vi "Pressure_1_R3.vi"() -> ()   [LabVIEW 2020]
uses:
  Support/Controls/Cmd_Mouse Popup.ctl
  Support/Controls/Clst_Initialize Input.ctl
  Support/Controls/Cmd_Var Data IO.ctl
  Variables/Global_Cal Info.vi
panel:
  in  "Measured_ADJ":string[][](table) caption="Measured (조정후)"
  out "최소용량":string
  out "분동조합":string[][](table)
  out "Form":string[][](table)
  in  "교정방법":string(combo)="기본교정"
  out "Resolution":string[][](table) caption="Spec"
  in  "지시형태":string(combo)="Check"
  in  "Spec 변경":bool
  in  "Random":bool
  out "Spec":string[][](table)
  out "제목":string
  out "에러 출력":errorcluster
  out "Condition":string[][](table)
  in  "최소눈금":string(combo)
  out "단위":string
  out "최대용량":string
  in  "Measured":string[][](table)
  out "Load?":bool
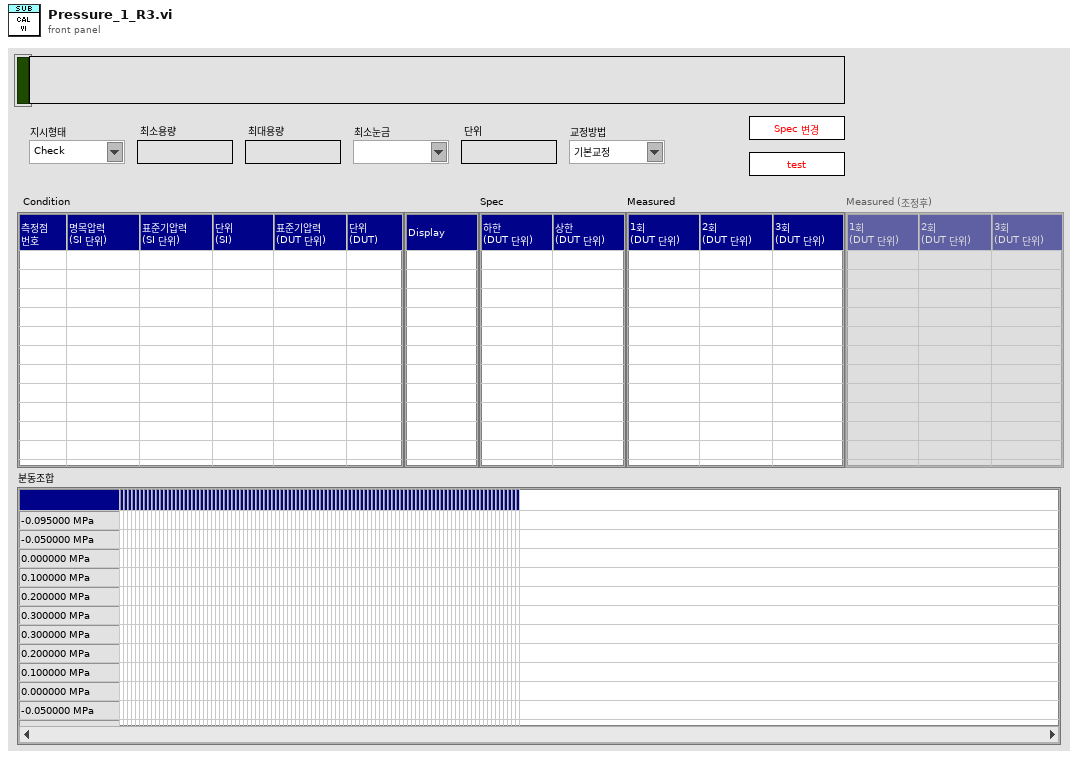
[diagram p1: front panel]
types:
  T1 = typedef "Cmd_Mouse Popup.ctl" = enum16{"활성화", "메뉴선택"}
  T2 = cluster{"Shift":bool, "Ctrl":bool, "Alt":bool, "Cmd":bool, "Opt":bool}
  T3 = typedef "Clst_Initialize Input.ctl" = cluster{"Initialize 1":cluster{"Condition":refnum<vi>[], "Spec":refnum<vi>[], "Measured":refnum<vi>[], "Resolution":refnum<vi>[], "Func_ext":string, "제목":refnum<vi>, "Measured_ADJ":refnum<vi>[]}, "Initialize 2":cluster{"문자열":refnum<vi>[], "콤보박스":refnum<vi>[], "링":refnum<vi>[], "열거형":refnum<vi>[], "테이블":refnum<vi>[], "여러열":refnum<vi>[], "디지털(DBL)":refnum<vi>[], "3D string":refnum<vi>[], "ctrl":refnum<vi>[], "boolean":refnum<vi>[]}}
  T4 = typedef "Cmd_Var Data IO.ctl" = enum16{"Condition", "Condition Default", "Condition_Temp", "Resolution", "Resolution Default", "Resolution Old", "Spec", "Spec Default", "Spec Old", "Spec Temp", "Result", "Result2", "Result3", "Result_Temp", "Result_ADJ", "Result_ADJ2", "STD1", "STD2", "STD3", "STD4", "STD5", "STD Temp", "CMC", "CMC Default"}
  T5 = enum8{"Enabled", "Disabled", "Disabled and Grayed Out"}
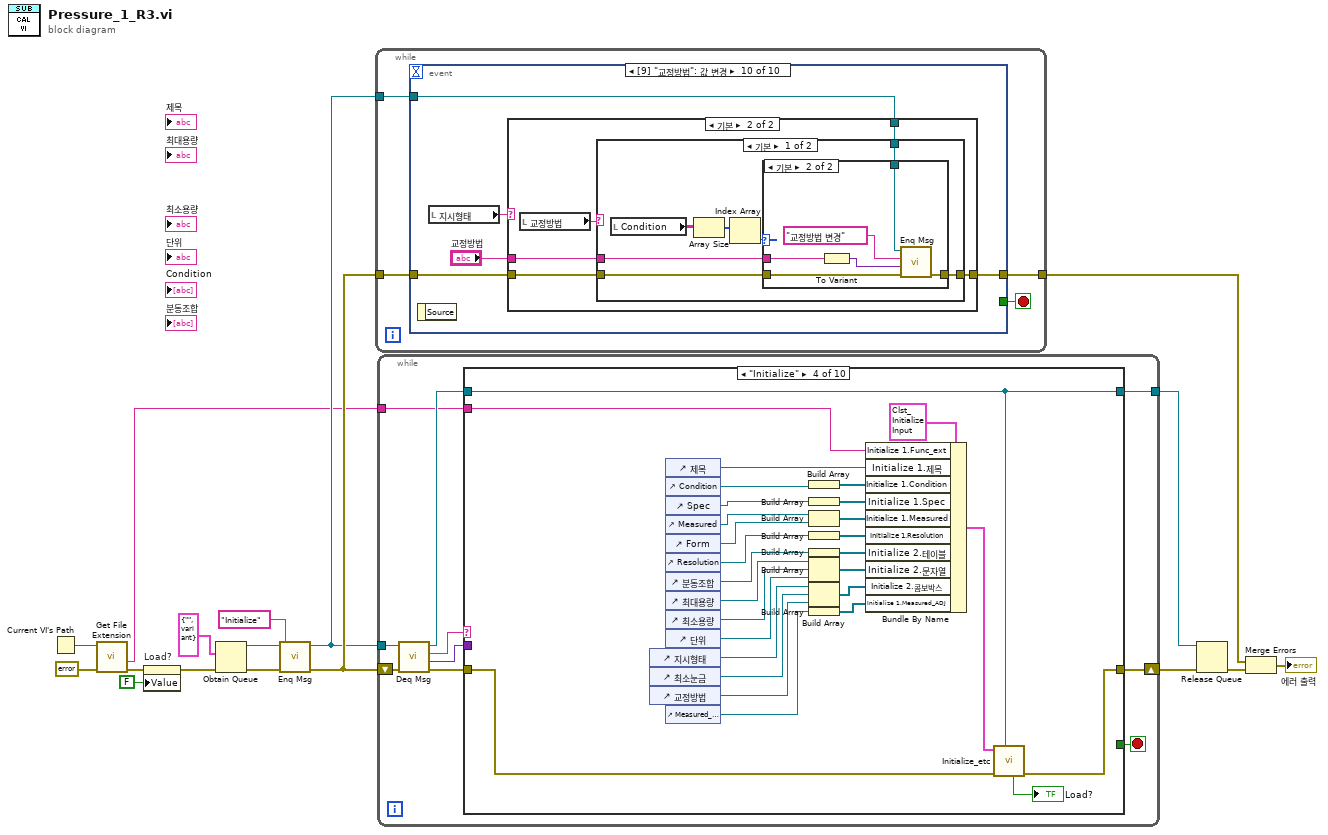
[diagram p0: block diagram]
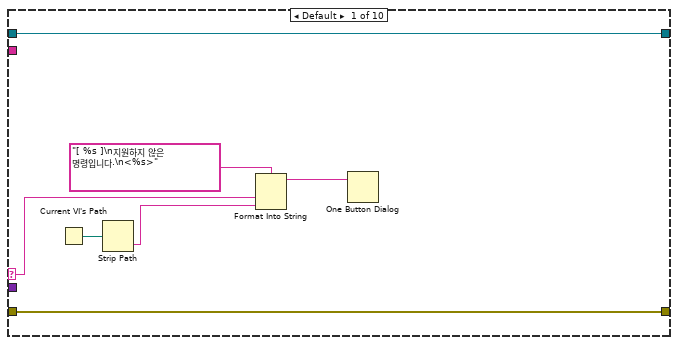
[diagram p2: hidden frame]
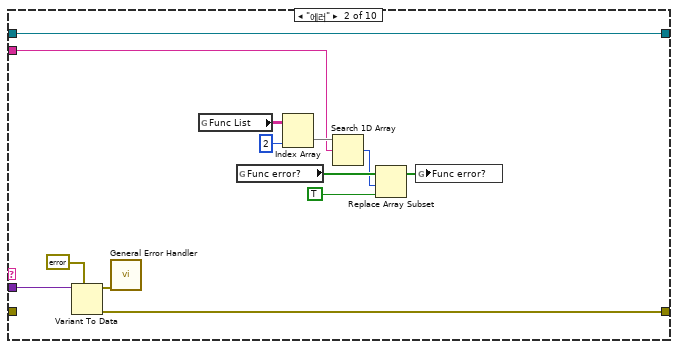
[diagram p3: hidden frame]
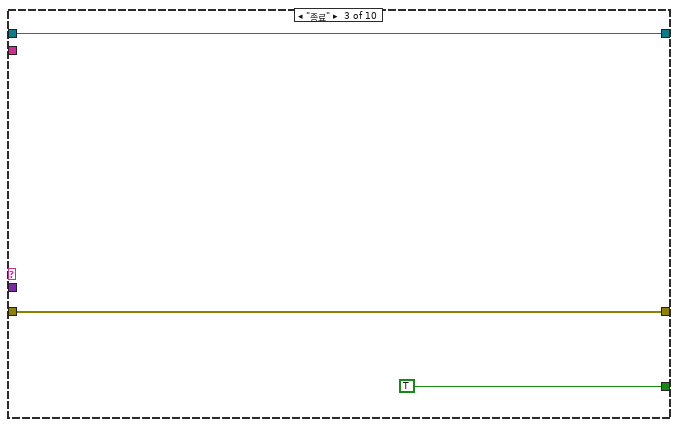
[diagram p4: hidden frame]
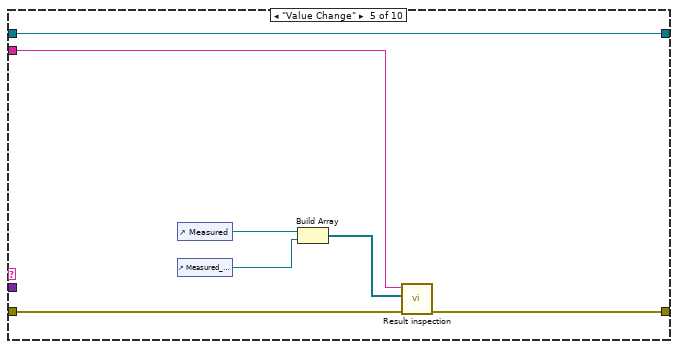
[diagram p5: hidden frame]
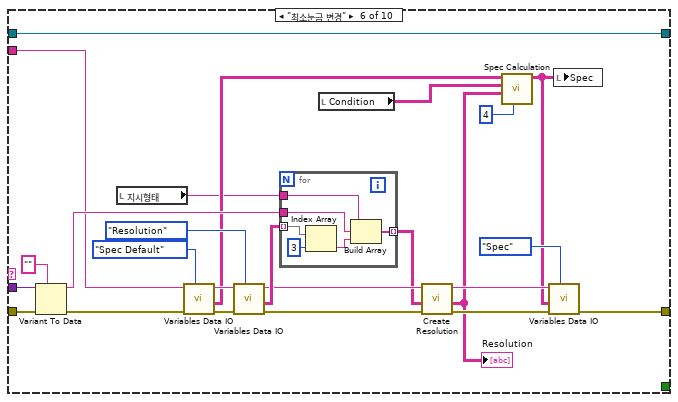
[diagram p6: hidden frame]
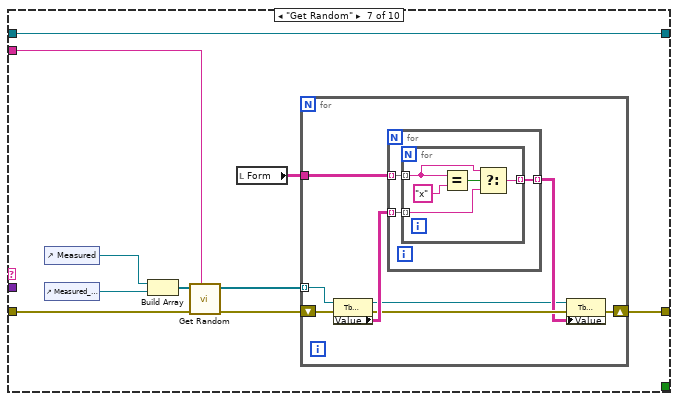
[diagram p7: hidden frame]
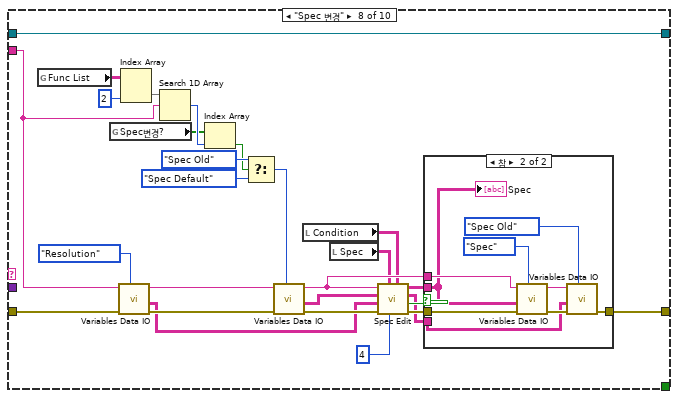
[diagram p8: hidden frame]
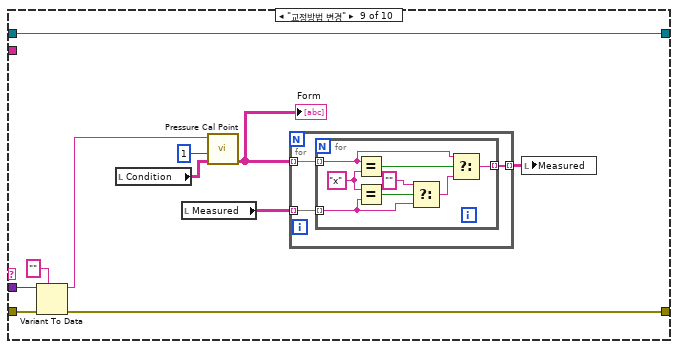
[diagram p10: hidden frame]
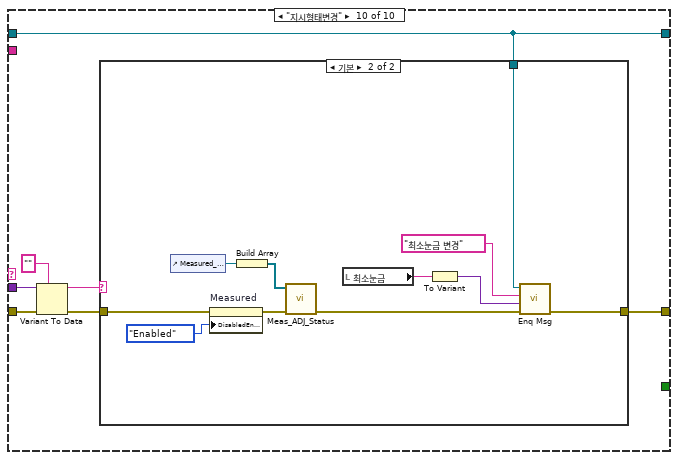
[diagram p11: hidden frame]
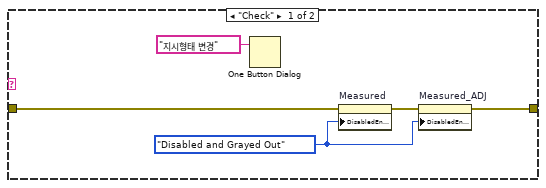
[diagram p12: hidden frame]
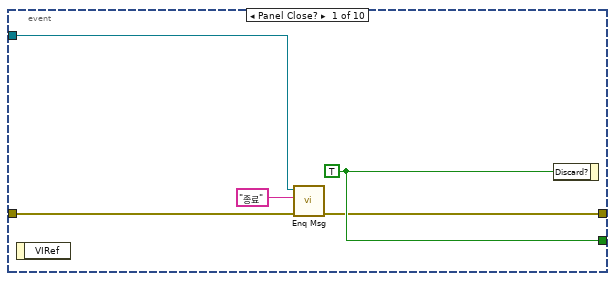
[diagram p13: hidden frame]
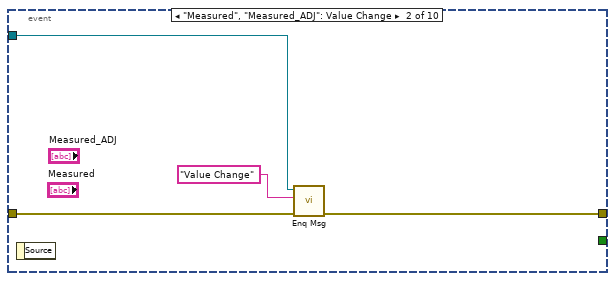
[diagram p14: hidden frame]
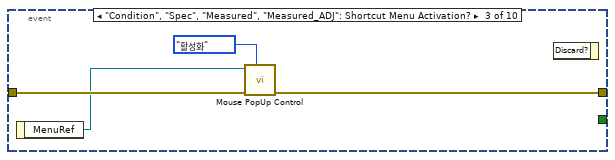
[diagram p15: hidden frame]
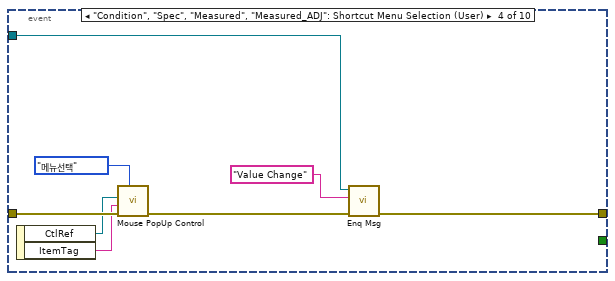
[diagram p16: hidden frame]
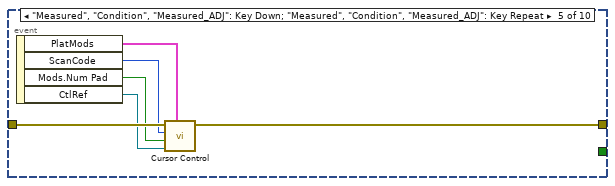
[diagram p17: hidden frame]
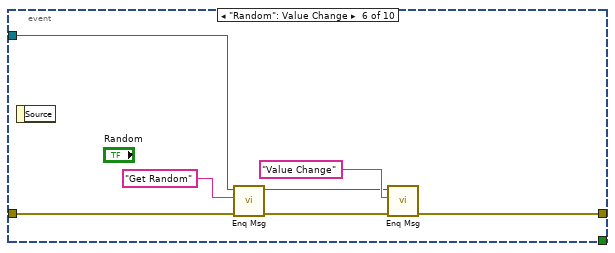
[diagram p18: hidden frame]
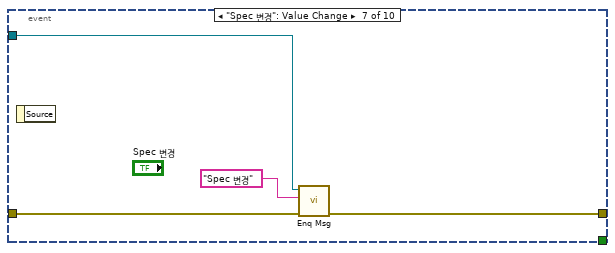
[diagram p19: hidden frame]
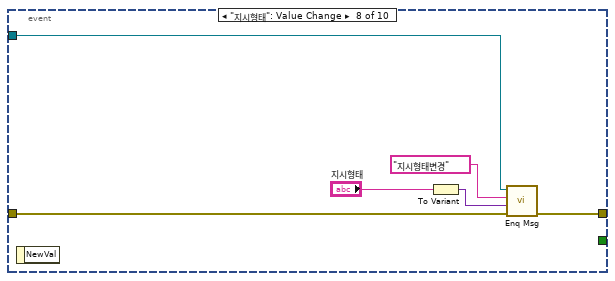
[diagram p20: hidden frame]
diagram:
  n1 = Current VI's Path() -> (path=w5:path)
  n2 = call <vilib>:"Get File Extension.vi"("error in (no error)"=errorcluster {"status"=FALSE, "code"=0, "source"=""} ("에러 상수"), "file"=w5) -> ("error out"=w3:errorcluster, "filename without extension"=w4:string)  [unwired: 5 in, 3 out]
  n3 = property on="Load?" class="Bool (엄격한)"(error in=w3, "Value"=FALSE ("Load?")) -> (error out=w2:errorcluster)  [unwired: 1 in, 1 out]
  n4 = Obtain Queue(element data type=cluster{"메세지":string, "값":variant} {"메세지"="", "값"=variant} ("Message Cluster"), error in (no error)=w2) -> (queue out=w14:refnum<queue>, error out=w16:errorcluster)  [unwired: 3 in, 1 out]
  n5 = call "Enq Msg.vi"("에러 입력(에러 없음)"=w16, "메세지"="Initialize", "큐 입력"=w14) -> ("에러 출력"=w15:errorcluster, "큐 출력"=w12:refnum<queue>)  [unwired: 7 in]
  n6 = while {
    tunnel: w15 -> [w19]
    tunnel: w12 -> [w20]
    tunnel: [w18] -> w9
    stop <- w21 stop-if-true
    n7 = event shown="[9] \"교정방법\": 값 변경" {
      selector: _ -> [_ _ _ _ _ _ _ _ _ _]
      dyn-events: _ -> [_ _ _ _ _ _ _ _ _ _]
      timeout: _ -> [_ _ _ _ _ _ _ _ _ _]
      tunnel: [w26 _ _ _ _ _ _ _ _ _] -> w21
      tunnel: w20 -> [w24 w29 _ w37 _ w50 w56 w62 w70 w72]
      tunnel: w19 -> [w25 w30 w33 w41 w48 w51 w58 w64 w71 w75]
      tunnel: [w22 w28 w32 w36 w47 w49 w57 w63 w69 w76] -> w18
      event Panel Close? {
        w26 = TRUE ("버림?")
        n8 = event-data() -> ()  [unwired: 1 in, 1 out]
        n9 = call "Enq Msg.vi"("에러 입력(에러 없음)"=w25, "메세지"="종료", "큐 입력"=w24) -> ("에러 출력"=w22:errorcluster)  [unwired: 7 in, 1 out]
        n10 = event-data("Discard?"=w26) -> ()  [unwired: 1 in, 1 out]
      }
      event "Measured", "Measured_ADJ": Value Change {
        n11 = event-data() -> ()  [unwired: 1 in, 1 out]
        n12 = call "Enq Msg.vi"("에러 입력(에러 없음)"=w30, "메세지"="Value Change", "큐 입력"=w29) -> ("에러 출력"=w28:errorcluster)  [unwired: 7 in, 1 out]
      }
      event "Condition", "Spec", "Measured", "Measured_ADJ": Shortcut Menu Activation? {
        n13 = event-data() -> ("MenuRef"=w31:refnum<k9>)  [unwired: 1 in]
        n14 = call "Mouse PopUp Control.vi"("type"=Cmd_Mouse_Popup."활성화", "error in"=w33, "메뉴 참조"=w31) -> ("error out"=w32:errorcluster)  [unwired: 8 in]
        n15 = event-data() -> ()  [unwired: 2 in, 1 out]
      }
      event "Condition", "Spec", "Measured", "Measured_ADJ": Shortcut Menu Selection (User) {
        n16 = event-data() -> ("CtlRef"=w39:refnum<vi>, "ItemTag"=w40:string)  [unwired: 1 in]
        n17 = call "Mouse PopUp Control.vi"("type"=Cmd_Mouse_Popup."메뉴선택", "error in"=w41, "아이템 태그"=w40, "Tbl 참조 번호"=w39) -> ("error out"=w38:errorcluster)  [unwired: 7 in]
        n18 = call "Enq Msg.vi"("에러 입력(에러 없음)"=w38, "메세지"="Value Change", "큐 입력"=w37) -> ("에러 출력"=w36:errorcluster)  [unwired: 7 in, 1 out]
      }
      event "Measured", "Condition", "Measured_ADJ": Key Down; "Measured", "Condition", "Measured_ADJ": Key Repeat {
        n19 = event-data() -> ("PlatMods"=w43:T2, "ScanCode"=w46:i16, "Mods.Num Pad"=w45:bool, "CtlRef"=w44:refnum<vi>)  [unwired: 1 in]
        n20 = call "Cursor Control.vi"("플랫폼 조합키"=w43, "참조"=w44, "Num Pad"=w45, "ScanCode"=w46, "error in"=w48) -> ("error out"=w47:errorcluster)  [unwired: 5 in, 1 out]
      }
      event "Random": Value Change {
        n21 = event-data() -> ()  [unwired: 1 in, 1 out]
        n22 = call "Enq Msg.vi"("에러 입력(에러 없음)"=w51, "메세지"="Get Random", "큐 입력"=w50) -> ("에러 출력"=w53:errorcluster, "큐 출력"=w54:refnum<queue>)  [unwired: 7 in]
        n23 = call "Enq Msg.vi"("에러 입력(에러 없음)"=w53, "메세지"="Value Change", "큐 입력"=w54) -> ("에러 출력"=w49:errorcluster)  [unwired: 7 in, 1 out]
      }
      event "Spec 변경": Value Change {
        n24 = event-data() -> ()  [unwired: 1 in, 1 out]
        n25 = call "Enq Msg.vi"("에러 입력(에러 없음)"=w58, "메세지"="Spec 변경", "큐 입력"=w56) -> ("에러 출력"=w57:errorcluster)  [unwired: 7 in, 1 out]
      }
      event "지시형태": Value Change {
        n26 = event-data() -> ()  [unwired: 1 in, 1 out]
        n27 = To Variant(anything="지시형태") -> (Variant=w60:variant)
        n28 = call "Enq Msg.vi"("에러 입력(에러 없음)"=w64, "값"=w60, "메세지"="지시형태변경", "큐 입력"=w62) -> ("에러 출력"=w63:errorcluster)  [unwired: 6 in, 1 out]
      }
      event "최소눈금": Value Change {
        n29 = event-data() -> ()  [unwired: 1 in, 1 out]
        n30 = To Variant(anything="최소눈금") -> (Variant=w66:variant)
        n31 = call "Enq Msg.vi"("에러 입력(에러 없음)"=w71, "값"=w66, "메세지"="최소눈금 변경", "큐 입력"=w70) -> ("에러 출력"=w69:errorcluster)  [unwired: 6 in, 1 out]
      }
      event "교정방법": Value Change {
        n32 = event-data() -> ()  [unwired: 1 in, 1 out]
        n33 = local read "지시형태"() -> (w73:string)
        n34 = case shown="기본" w73 {
          tunnel: w75 -> [w78 w83]
          tunnel: w72 -> [_ w82]
          tunnel: [w78 w81] -> w76
          tunnel: "교정방법" -> [_ w80]
          frame "Check" {
            n35 = One Button Dialog(message="지시형태 변경" ("메시지")) -> ()  [unwired: 1 in, 1 out]
          }
          frame Default {
            n36 = local read "교정방법"() -> (w79:string)
            n37 = case shown="기본" w79 {
              tunnel: w83 -> [w90 w105]
              tunnel: w82 -> [w89 w104]
              tunnel: [w88 w103] -> w81
              tunnel: w80 -> [w87 w102]
              frame Default {
                n38 = local read "Condition"() -> (w84:string[][])
                n39 = Array Size(array=w84) -> (size(s)=w86:i32[])
                n40 = Index Array(array=w86) -> (element=w85:i32)  [unwired: 1 in]
                n41 = case shown="기본" w85 {
                  tunnel: w90 -> [w93 w99]
                  tunnel: w89 -> [_ w98]
                  tunnel: [w93 w96] -> w88
                  tunnel: w87 -> [_ w94]
                  frame 0..21 {
                    n42 = local write "교정방법"("기본교정" ("교정방법")) -> ()
                    n43 = One Button Dialog(message="표준, 종합 교정은 11 측정점 이상 가능" ("메시지")) -> ()  [unwired: 1 in, 1 out]
                  }
                  frame Default {
                    n44 = To Variant(anything=w94) -> (Variant=w95:variant)
                    n45 = call "Enq Msg.vi"("에러 입력(에러 없음)"=w99, "값"=w95, "메세지"="교정방법 변경", "큐 입력"=w98) -> ("에러 출력"=w96:errorcluster)  [unwired: 6 in, 1 out]
                  }
                }
              }
              frame "기본교정" {
                n46 = To Variant(anything=w102) -> (Variant=w100:variant)
                n47 = call "Enq Msg.vi"("에러 입력(에러 없음)"=w105, "값"=w100, "메세지"="교정방법 변경", "큐 입력"=w104) -> ("에러 출력"=w103:errorcluster)  [unwired: 6 in, 1 out]
              }
            }
          }
        }
      }
    }
  }
  n48 = while {
    shift-right: [w115] -> w11
    shift-left: w15 -> [w114]
    tunnel: w12 -> [w112]
    tunnel: [w107] -> w10
    tunnel: w4 -> [w106]
    stop <- w108 stop-if-true
    n49 = call "Deq Msg.vi"("에러 입력(에러 없음)"=w114, "큐 입력"=w112) -> ("에러 출력"=w113:errorcluster, "값"=w109:variant, "메세지"=w111:string, "큐 출력"=w110:refnum<queue>)  [unwired: 6 in]
    n50 = case shown="\"Initialize\"" w111 {
      selector: w111 -> [w118 _ _ _ _ _ _ _ _ _]
      tunnel: w113 -> [w122 _ w138 w151 w171 w197 w213 w252 w276 w296]
      tunnel: [w122 w132 w138 w140 w173 w179 w208 w256 w275 w297] -> w115
      tunnel: w110 -> [w121 w131 w136 w152 w174 w199 w215 w258 w279 w291]
      tunnel: w109 -> [_ w133 _ _ _ w196 _ _ w277 w294]
      tunnel: [_ _ TRUE ("버림?") _ _ _ _ _ _ _] -> w108
      tunnel: [w121 w131 w136 w152 w174 w199 w215 w258 w279 w291] -> w107
      tunnel: w106 -> [_ w123 _ w144 w172 w189 w211 w233 _ _]
      frame Default {
        n51 = Current VI's Path() -> (path=w117:path)
        n52 = Strip Path(path=w117) -> (name=w116:string)  [unwired: 1 out]
        n53 = Format Into String(format string="[ %s ]\n지원하지 않은 명령입니다.\n<%s>" ("메시지"), w118, w116) -> (resulting string=w119:string)  [unwired: 2 in, 1 out]
        n54 = One Button Dialog(message=w119) -> ()  [unwired: 1 in, 1 out]
      }
      frame "에러" {
        n55 = Variant To Data(type=errorcluster {"status"=FALSE, "code"=0, "source"=""} ("에러 출력"), Variant=w133) -> (data=w135:errorcluster, error out=w132:errorcluster)  [unwired: 1 in]
        n56 = call <vilib>:"General Error Handler.vi"("error in (no error)"=w135) -> ()  [unwired: 10 in, 5 out]
        n57 = global read "Global_Cal Info.vi" "Func List"() -> (w129:string[][])
        n58 = global read "Global_Cal Info.vi" "Func error?"() -> (w126:bool[])
        n59 = Index Array(array=w129, index (col)=2 ("비활성화된 인덱스 (열)")) -> (element=w128:string[])  [unwired: 1 in]
        n60 = Search 1D Array(1D array=w128, element=w123) -> (index of element=w125:i32)  [unwired: 1 in]
        n61 = Replace Array Subset(array=w126, new element=TRUE ("새 원소/부분배열"), index=w125) -> (w124:bool[])
        n62 = global write "Global_Cal Info.vi" "Func error?"(w124) -> ()
      }
      frame "종료" {
      }
      frame "Initialize" {
        n63 = control-ref of="지시형태"() -> (w147:refnum<vi>)
        n64 = control-ref of="최소눈금"() -> (w159:refnum<vi>)
        n65 = control-ref of="교정방법"() -> (w146:refnum<vi>)
        n66 = control-ref of="제목"() -> (w157:refnum<vi>)
        n67 = control-ref of="Condition"() -> (w165:refnum<vi>)
        n68 = control-ref of="Spec"() -> (w154:refnum<vi>)
        n69 = control-ref of="Measured"() -> (w162:refnum<vi>)
        n70 = control-ref of="Form"() -> (w145:refnum<vi>)
        n71 = control-ref of="Resolution"() -> (w149:refnum<vi>)
        n72 = control-ref of="분동조합"() -> (w150:refnum<vi>)
        n73 = control-ref of="최대용량"() -> (w156:refnum<vi>)
        n74 = control-ref of="최소용량"() -> (w143:refnum<vi>)
        n75 = control-ref of="단위"() -> (w155:refnum<vi>)
        n76 = control-ref of="Measured_ADJ"() -> (w142:refnum<vi>)
        n77 = Build Array(w165) -> (w164:refnum<vi>[])
        n78 = Build Array(w154) -> (w153:refnum<vi>[])
        n79 = Build Array(w162, w145) -> (w163:refnum<vi>[])
        n80 = Build Array(w149) -> (w148:refnum<vi>[])
        n81 = Build Array(w150) -> (w161:refnum<vi>[])
        n82 = Build Array(w156, w143, w155) -> (w160:refnum<vi>[])
        n83 = Build Array(w147, w159, w146) -> (w158:refnum<vi>[])
        n84 = Build Array(w142) -> (w141:refnum<vi>[])
        n85 = Bundle By Name(cluster=T3 {"Initialize 1"={"Condition"=[], "Spec"=[], "Measured"=[], "Resolution"=[], "Func_ext"="", "제목"=refnum, "Measured_ADJ"=[]}, "Initialize 2"={"문자열"=[], "콤보박스"=[], "링"=[], "열거형"=[], "테이블"=[], "여러열"=[], "디지털(DBL)"=[], "3D string"=[], "ctrl"=[], "boolean"=[]}} ("입력 클러스터"), "Initialize 1.Func_ext"=w144, "Initialize 1.제목"=w157, "Initialize 1.Condition"=w164, "Initialize 1.Spec"=w153, "Initialize 1.Measured"=w163, "Initialize 1.Resolution"=w148, "Initialize 2.테이블"=w161, "Initialize 2.문자열"=w160, "Initialize 2.콤보박스"=w158, "Initialize 1.Measured_ADJ"=w141) -> (w166:T3)
        n86 = call "Initialize_etc.vi"("큐 입력"=w152, "error in"=w151, "입력 클러스터"=w166) -> ("error out"=w140:errorcluster, "Load?"=→"Load?":bool)  [unwired: 6 in, 1 out]
      }
      frame "Value Change" {
        n87 = control-ref of="Measured"() -> (w170:refnum<vi>)
        n88 = control-ref of="Measured_ADJ"() -> (w168:refnum<vi>)
        n89 = Build Array(w170, w168) -> (w169:refnum<vi>[])
        n90 = call "Result inspection.vi"("error in"=w171, "Ref. Data (Inspection)"=w169, "Func ext"=w172) -> ("error out"=w173:errorcluster)  [unwired: 5 in, 3 out]
      }
      frame "최소눈금 변경" {
        n91 = Variant To Data(error in=w197, type="", Variant=w196) -> (data=w194:string, error out=w190:errorcluster)
        n92 = local read "지시형태"() -> (w175:string)
        n93 = call "Variables Data IO.vi"("Select"=Cmd_Var_Data_IO."Spec Default", "error in"=w190, "Func_ext"=w189) -> ("error out"=w187:errorcluster, "Data Out"=w185:string[][], "Func_ext Out"=w188:string)  [unwired: 6 in]
        n94 = call "Variables Data IO.vi"("Select"=Cmd_Var_Data_IO."Resolution", "error in"=w187, "Func_ext"=w188) -> ("error out"=w192:errorcluster, "Data Out"=w198:string[][], "Func_ext Out"=w191:string)  [unwired: 6 in]
        n95 = for {
          tunnel: w198 -> [w205] mode=indexing
          tunnel: w194 -> [w204]
          tunnel: [w202] -> w177 mode=indexing
          tunnel: w175 -> [w201]
          n96 = Index Array(array=w205, index=3 ("인덱스")) -> (element=w203:string)
          n97 = Build Array(w201, w204, w203) -> (w202:string[])
        }
        n98 = local read "Condition"() -> (w184:string[][])
        n99 = call "Create Resolution.vi"("에러 입력(에러 없음)"=w192, "Resolution"=w177, "Func_ext"=w191) -> ("에러 출력"=w180:errorcluster, "Resolution Out"=w176:string[][], "Func_ext 출력"=w181:string)  [unwired: 6 in]
        "Resolution" <- w176
        n100 = call "Spec Calculation.vi"("기준값 열번호"=4 ("열번호(기준값)"), "Resolution"=w176, "Condition in"=w184, "Spec Default"=w185) -> ("Spec out"=w178:string[][])  [unwired: 6 in, 1 out]
        n101 = call "Variables Data IO.vi"("Select"=Cmd_Var_Data_IO."Spec", "error in"=w180, "Data In"=w178, "Func_ext"=w181) -> ("error out"=w179:errorcluster)  [unwired: 5 in, 2 out]
        n102 = local write "Spec"(w178) -> ()
      }
      frame "Get Random" {
        n103 = control-ref of="Measured"() -> (w212:refnum<vi>)
        n104 = control-ref of="Measured_ADJ"() -> (w210:refnum<vi>)
        n105 = Build Array(w212, w210) -> (w214:refnum<vi>[])
        n106 = call "Get Random.vi"("Func_Ext"=w211, "에러 입력"=w213, "Meas"=w214) -> ("에러 출력"=w209:errorcluster, "Meas out"=w206:refnum<vi>[])  [unwired: 7 in]
        n107 = local read "Form"() -> (w207:string[][])
        n108 = for {
          tunnel: w207 -> [w222]
          shift-right: [w219] -> w208
          shift-left: w209 -> [w223]
          tunnel: w206 -> [w216] mode=indexing
          n109 = property on="프로퍼티 노드" class="Tbl (엄격한)"(reference=w216, error in=w223) -> (reference out=w217:refnum<vi>, error out=w220:errorcluster, "Value"=w221:string[][])
          n110 = for {
            tunnel: w222 -> [w226] mode=indexing
            tunnel: w221 -> [w225] mode=indexing
            tunnel: [w224] -> w218 mode=indexing
            n111 = for {
              tunnel: w226 -> [w229] mode=indexing
              tunnel: w225 -> [w228] mode=indexing
              tunnel: [w227] -> w224 mode=indexing
              n112 = Equal?(x=w229, y="ⅹ") -> (x = y?=w230:bool)
              n113 = Select(t=w229, s=w230, f=w228) -> (s? t:f=w227:string)
            }
          }
          n114 = property on="프로퍼티 노드" class="Tbl (엄격한)"(reference=w217, error in=w220, "Value"=w218) -> (error out=w219:errorcluster)  [unwired: 1 out]
        }
      }
      frame "Spec 변경" {
        n115 = global read "Global_Cal Info.vi" "Func List"() -> (w238:string[][])
        n116 = global read "Global_Cal Info.vi" "Spec변경?"() -> (w234:bool[])
        n117 = call "Variables Data IO.vi"("Select"=Cmd_Var_Data_IO."Resolution", "error in"=w252, "Func_ext"=w233) -> ("error out"=w251:errorcluster, "Data Out"=w245:string[][], "Func_ext Out"=w250:string)  [unwired: 6 in]
        n118 = Index Array(array=w238, index (col)=2 ("비활성화된 인덱스 (열)")) -> (element=w236:string[])  [unwired: 1 in]
        n119 = Search 1D Array(1D array=w236, element=w233) -> (index of element=w235:i32)  [unwired: 1 in]
        n120 = Index Array(array=w234, index=w235) -> (element=w239:bool)
        n121 = Select(t=Cmd_Var_Data_IO."Spec Old" ("Select"), s=w239, f=Cmd_Var_Data_IO."Spec Default" ("Select")) -> (s? t:f=w232:T4)
        n122 = call "Variables Data IO.vi"("Select"=w232, "error in"=w251, "Func_ext"=w250) -> ("error out"=w253:errorcluster, "Data Out"=w244:string[][], "Func_ext Out"=w246:string)  [unwired: 6 in]
        n123 = local read "Condition"() -> (w242:string[][])
        n124 = local read "Spec"() -> (w243:string[][])
        n125 = call "Spec Edit.vi"("Condition"=w242, "열번호(기준값)"=4 ("기준열(0)"), "Spec Value"=w243, "에러 입력(에러 없음)"=w253, "Resolution"=w245, "Spec Default"=w244, "Func_ext"=w246) -> ("에러 출력"=w257:errorcluster, "변경?"=w254:bool, "Spec Default out"=w248:string[][], "Spec 출력"=w255:string[][])  [unwired: 1 in]
        n126 = case shown="참" w254 {
          tunnel: w257 -> [w259 w267]
          tunnel: [w259 w263] -> w256
          tunnel: w255 -> [_ w265]
          tunnel: w246 -> [_ w266]
          tunnel: w248 -> [_ w261]
          frame False {
          }
          frame True {
            n127 = call "Variables Data IO.vi"("Select"=Cmd_Var_Data_IO."Spec", "error in"=w267, "Data In"=w265, "Func_ext"=w266) -> ("error out"=w264:errorcluster, "Func_ext Out"=w262:string)  [unwired: 5 in, 1 out]
            n128 = call "Variables Data IO.vi"("Select"=Cmd_Var_Data_IO."Spec Old", "error in"=w264, "Data In"=w261, "Func_ext"=w262) -> ("error out"=w263:errorcluster)  [unwired: 5 in, 2 out]
            "Spec" <- w265
          }
        }
      }
      frame "교정방법 변경" {
        n129 = Variant To Data(error in=w276, type="", Variant=w277) -> (data=w272:string, error out=w275:errorcluster)
        n130 = local read "Condition"() -> (w271:string[][])
        n131 = local read "Measured"() -> (w274:string[][])
        n132 = call "Pressure Cal Point.vi"("Condition"=w271, "인덱스 (열)"=1, "교정방법"=w272) -> ("배열"=w269:string[][])  [unwired: 5 in, 3 out]
        "Form" <- w269
        n133 = for {
          tunnel: w269 -> [w282] mode=indexing
          tunnel: w274 -> [w281] mode=indexing
          tunnel: [w280] -> w273 mode=indexing
          n134 = for {
            tunnel: w282 -> [w289] mode=indexing
            tunnel: w281 -> [w285] mode=indexing
            tunnel: [w283] -> w280 mode=indexing
            w288 = "ⅹ"
            n135 = Equal?(x=w289, y=w288) -> (x = y?=w290:bool)
            n136 = Equal?(x=w288, y=w285) -> (x = y?=w287:bool)
            n137 = Select(t="", s=w287, f=w285) -> (s? t:f=w284:string)
            n138 = Select(t=w289, s=w290, f=w284) -> (s? t:f=w283:string)
          }
        }
        n139 = local write "Measured"(w273) -> ()
      }
      frame "지시형태변경" {
        n140 = Variant To Data(error in=w296, type="", Variant=w294) -> (data=w292:string, error out=w295:errorcluster)
        n141 = case shown="기본" w292 {
          tunnel: w295 -> [w301 w312]
          tunnel: [w298 w305] -> w297
          tunnel: w291 -> [_ w303]
          frame "Check" {
            w300 = T5."Disabled and Grayed Out" ("비활성화")
            n142 = One Button Dialog(message="지시형태 변경" ("메시지")) -> ()  [unwired: 1 in, 1 out]
            n143 = property on="Measured" class="Tbl (엄격한)"(error in=w301, "DisabledEnum"=w300) -> (error out=w299:errorcluster)  [unwired: 1 in, 1 out]
            n144 = property on="Measured_ADJ" class="Tbl (엄격한)"(error in=w299, "DisabledEnum"=w300) -> (error out=w298:errorcluster)  [unwired: 1 in, 1 out]
          }
          frame Default {
            n145 = control-ref of="Measured_ADJ"() -> (w311:refnum<vi>)
            n146 = property on="Measured" class="Tbl (엄격한)"(error in=w312, "DisabledEnum"=T5."Enabled" ("비활성화")) -> (error out=w309:errorcluster)  [unwired: 1 in, 1 out]
            n147 = Build Array(w311) -> (w310:refnum<vi>[])
            n148 = call "Meas_ADJ_Status.vi"("에러 입력(에러 없음)"=w309, "Measured_ADJ in"=w310) -> ("에러 출력"=w306:errorcluster)  [unwired: 8 in, 1 out]
            n149 = local read "최소눈금"() -> (w304:string)
            n150 = To Variant(anything=w304) -> (Variant=w308:variant)
            n151 = call "Enq Msg.vi"("에러 입력(에러 없음)"=w306, "값"=w308, "메세지"="최소눈금 변경", "큐 입력"=w303) -> ("에러 출력"=w305:errorcluster)  [unwired: 6 in, 1 out]
          }
        }
      }
    }
  }
  n152 = Release Queue(queue=w10, error in (no error)=w11) -> (error out=w8:errorcluster)  [unwired: 1 in, 2 out]
  n153 = Merge Errors(w9, w8) -> (→"에러 출력":errorcluster)
